vi "Dashboard Main1920x1080fixed.vi"() -> ()   [LabVIEW 2025]
uses:
  <vilib>/event_ctls.llb/eventvkey.ctl
  DashBoardGlobals.vi
  <vilib>/Rock Robotics/Network Tables/NT Read Numeric Array.vi
  <vilib>/Rock Robotics/WPI/Dashboard/WPI_DashboardLogging Global.vi
panel:
  in  "TCP":refnum<k5>
  out "Vision/Cam4Orientation":dbl caption="Cam 1 Yaw" format="%11.2f"
  out "Vision/Cam4Z":dbl caption="Cam 1 Z" format="%11.2f"
  out "Vision/Cam4Y":dbl caption="Cam 1 Y" format="%11.2f"
  out "Vision/Cam4Count":dbl caption="Cam1 Count" format="%13.0f"
  out "Vision/Cam4X":dbl caption="Cam 1 X" format="%11.2f"
  out "Vision/Cam3Orientation":dbl caption="Cam 1 Yaw" format="%11.2f"
  out "Vision/Cam3Z":dbl caption="Cam 1 Z" format="%11.2f"
  out "Vision/Cam3Y":dbl caption="Cam 1 Y" format="%11.2f"
  out "Vision/Cam3Count":dbl caption="Cam1 Count" format="%13.0f"
  out "Vision/Cam3X":dbl caption="Cam 1 X" format="%11.2f"
  out "Vision/Cam2Orientation":dbl caption="Cam 1 Yaw" format="%11.2f"
  out "Vision/Cam2Z":dbl caption="Cam 1 Z" format="%11.2f"
  out "Vision/Cam2Y":dbl caption="Cam 1 Y" format="%11.2f"
  out "Vision/Cam2Count":dbl caption="Cam1 Count" format="%13.0f"
  out "Vision/Cam2X":dbl caption="Cam 1 X" format="%11.2f"
  out "Vision/Cam1Orientation":dbl caption="Cam 1 Yaw" format="%11.2f"
  out "Vision/Cam1Z":dbl caption="Cam 1 Z" format="%11.2f"
  out "Vision/Cam1Y":dbl caption="Cam 1 Y" format="%11.2f"
  out "Vision/Cam1Count":dbl caption="Cam1 Count" format="%13.0f"
  out "Vision/Cam1X":dbl caption="Cam 1 X" format="%11.2f"
  out "NT Connection":bool
  out "Mode":T1(ring)=enum."Auto Disabled"
  out "BelowLeftCamBackground":bool
  in  "Camera Settings Right":T2={"Frame Rate"=30, "Compression"=30, "Size"=1, "DB Camera Config"=FALSE} {"Frame Rate" scale=1.0..30.0; "Compression" scale=100.0..-1.0; "Size" items=["640x480", "320x240", "160x120"]}
  in  "Camera Name Right":string(combo)="No Camera Selection"
  out "Camera Perf":string
  in  "Camera Settings":T2={"Frame Rate"=30, "Compression"=30, "Size"=1, "DB Camera Config"=FALSE} {"Frame Rate" scale=1.0..30.0; "Compression" scale=100.0..-1.0; "Size" items=["640x480", "320x240", "160x120"]}
  in  "Rec Mode":enum32{"Stop", "Record", "Playback"}(radio)
  out "Robot IP":string
  out "Image Message":string="Timeout in Camera Communications"
  in  "Dashboard Tab":T3(tab)
  out "MotorChart R":cluster{"Numeric":dbl, "Numeric":dbl}(graph)
  out "MotorChart L":cluster{"Numeric":dbl, "Numeric":dbl}(graph)
  out "MotorSliders R":cluster{"MotorSlide1":dbl, "MotorSlide2":dbl} {"MotorSlide2" scale=-1.0..1.0 scale format="%#_2e"; "MotorSlide1" scale=-1.0..1.0 scale format="%#_2e"}
  out "MotorSliders L":cluster{"MotorSlide1":dbl, "MotorSlide2":dbl} {"MotorSlide2" scale=-1.0..1.0 scale format="%#_2e"; "MotorSlide1" scale=-1.0..1.0 scale format="%#_2e"}
  out "JS1 Z":dbl(slide) scale=-1.0..1.0 scale format="%#_2e"
  out "JS1 Graph":cluster{"X":dbl, "Y":dbl}[](graph)
  out "JS1 Buttons":T4
  out "JS2 Z":dbl(slide) scale=-1.0..1.0 scale format="%#_2e"
  out "JS2 Graph":cluster{"X":dbl, "Y":dbl}[](graph)
  out "JS2 Buttons":T4
  out "Gyro":dbl(knob) scale=0.0..360.0
  out "Right Camera Perf":cluster{"Bandwidth (Mbps)":dbl, "FPS":dbl}
  out "Camera Image Right":T5(plugin-control)
  out "TurretLauncher/LauncherOn":bool caption="Launcher On"
  out "TurretLauncher/LauncherManual":bool caption="Manual"
  out "TurretLauncher/LauncherSpeed2":dbl caption="Motor 2 Speed" format="%11.0f"
  out "TurretLauncher/LauncherSpeed1":dbl caption="Motor 1 Speed" format="%11.0f"
  out "TurretLauncher/LauncherSpeedActual":dbl caption="Average Speed RPM" format="%11.0f"
  out "TurretLauncher/LauncherMotorDmd":dbl caption="Motor Dmd" format="%11.2f"
  out "TurretLauncher/LauncherTargetSpeed":dbl caption="Desired Speed RPM" format="%11.0f"
  out "TurretLauncher/SpeedOnTarget":bool caption="On Target"
  out "Teleop/GoClimb":bool caption="GO CLIMB"
  out "Teleop/FieldOriented":bool caption="Field Oriented"
  out "MatchSystem/isRed":bool caption="Is Red"
  out "MatchSystem/isBlue":bool caption="Is Blue"
  out "TurretLauncher/TurretManualMode":bool caption="Manual"
  out "TurretLauncher/TurretEncoderRotation":dbl caption="Pos Deg" format="%12.1f"
  out "TurretLauncher/OnTarget":bool caption="On Target"
  out "TurretLauncher/TurretMotorDmd":dbl caption="Motor Output" format="%11.2f"
  out "TurretLauncher/TurretDesiredAngle":dbl caption="Pos Dmd Deg" format="%12.1f"
  out "TurretLauncher/TurretclockwiseLimitSwitch":bool caption="CW Limit"
  out "TurretLauncher/TurretcounterclockwiseLimitSwitch":bool caption="CCW Limit"
  out "IntakeSystem/IntakeAngleMotorDmd":dbl caption="Pos Motor Dmd" format="%11.2f"
  out "IntakeSystem/IntakeAngleTarget":dbl caption="Position Dmd Deg" format="%12.1f"
  out "IntakeSystem/IntakeMotorRPM":dbl caption="Intake RPM" format="%12.1f"
  out "IntakeSystem/IntakeMotorOut":dbl caption="Intake Motor Dmd" format="%11.2f"
  out "IntakeSystem/EncoderRotation":dbl caption="Position Act Deg" format="%12.1f"
  out "IntakeSystem/IntakeLimitIsPressed":bool caption="LowLimitSwitch"
  out "IntakeSystem/IntakeIsExtended":bool caption="Extended"
  out "Supervisory/Mode":string caption="Mode"
  out "AutoSystem/StepTime":dbl caption="Step Time" format="%11.2f"
  out "Auto Selector":string caption="Name"
  out "AutoSystem/Step":T6(ring) caption="Cmd Name"
  out "AutoSystem/function":string caption="Function"
  out "AutoSystem/Parm2":dbl caption="Parm 2" format="%11.2f"
  out "AutoSystem/Parm1":dbl caption="Parm 1" format="%11.2f"
  out "AutoSystem/Timeout":dbl caption="Time out Sec" format="%11.2f"
  out "AutoSystem/Parm3":dbl caption="Parm 3" format="%11.2f"
  out "AutoSystem/Step":dbl caption="Cmd" format="%13.0f"
  out "TrajectorySystem/done":bool caption="Done"
  out "TrajectorySystem/ElapsedTrajTime":dbl caption="Elapsed Time" format="%12.1f"
  out "TrajectorySystem/rotErr":dbl caption="Rotational Error" format="%11.2f"
  out "TrajectorySystem/yErr":dbl caption="Y Error" format="%11.2f"
  out "TrajectorySystem/timeLengthOfTrajectory":dbl caption="Total Time" format="%12.1f"
  out "TrajectorySystem/xErr":dbl caption="X Error" format="%11.2f"
  out "TrajectorySystem/onTarget":bool caption="On Target"
  out "SwerveDrive/omegaActual":dbl caption="Vel Rot" format="%11.2f"
  out "SwerveDrive/vyActual":dbl caption="Vel Y" format="%12.1f"
  out "SwerveDrive/vyTarget":dbl caption="Vel Y Dmd" format="%12.1f"
  out "SwerveDrive/vxActual":dbl caption="Vel X" format="%12.1f"
  out "SwerveDrive/vxTarget":dbl caption="Vel X Dmd" format="%12.1f"
  out "SwerveDrive/GyroYaw":dbl caption="Gyro Yaw" format="%12.1f"
  out "SwerveDrive/GyroRoll":dbl caption="Gyro Roll" format="%12.1f"
  out "SwerveDrive/omegaTarget":dbl caption="Vel Rot Dmd" format="%11.2f"
  out "SwerveDrive/GyroPitch":dbl caption="Gyro Pitch" format="%12.1f"
  out "SwerveDrive/GyroConnected":bool caption="Gyro Connected"
  out "FeederSystem/FeederRPM":dbl caption="Speed RPM" format="%12.1f"
  out "FeederSystem/FeederOutput":dbl caption="Motor Dmd" format="%11.2f"
  out "FeederSystem/FeederState":bool caption="Feeder On"
  out "AgitatorSystem/AgitatorRPM":dbl caption="Speed  RPM" format="%12.1f"
  out "AgitatorSystem/AgitatorOutput":dbl caption="Motor Dmd" format="%11.2f"
  out "AgitatorSystem/AgitatorState":bool caption="Agitator On"
  in  "Select Auto":string(combo)="Select Autonomous ..."
  out "Odometry/Rotation_position":dbl caption="Rotation Rad" format="%11.2f"
  out "Odometry/Y_position":dbl caption="Y Pos M" format="%11.2f"
  out "Odometry/execElapsedTime":dbl caption="Elapsed Time" format="%9.3f"
  out "Odometry/X_position":dbl caption="X Pos M" format="%11.2f"
  in  "Test Slider":dbl(slide) scale=0.0..100.0 scale format="%#_3g"
  in  "On/Off":bool caption="Solenoid"
  in  "Test Name":u16(ring) items=["Select the test to run..."]
  in  "Test Tree":string(tree)
  in  "Motor":cluster{"Value":dbl, "Enable":bool} {"Value" scale=-1.0..1.0 scale format="%#_3g"}
  out "Progress":T7 {"Test Progress" scale=0.0..100.0}
  in  "Rev/Fwd":cluster{"Forward":bool, "Reverse":bool}
  in  "Test Ring":u16(ring) items=["Monochrome", "Color"]
  in  "CheckList":i32(listbox)
  out "Tree":string(tree)
  out "Camera Image":T5(plugin-control)
  out "Background":bool
  in  "Camera Name":string(combo)="No Camera Selection"
  # "VISION"
  # "Cam 1"
  # "Cam 2"
  # "Cam 3"
  # "Cam 4"
  # "Count"
  # "X"
  # "Y"
  # "Z"
  # "Yaw"
  # "HW"
  # "HW"
  # "Drive Motors"
  # "Front"
  # "Right"
  # "Left"
  # "Back"
  # "Joysticks"
  # "LAUNCHER"
  # "TELEOP"
  # "MATCH"
  # "TURRET"
  # "INTAKE"
  # "SUPERVISORY"
  # "AUTO"
  # "TRAJECTORY"
  # "DRIVE"
  # "FEEDER"
  # "AGITATOR"
  # "ODOMETRY"
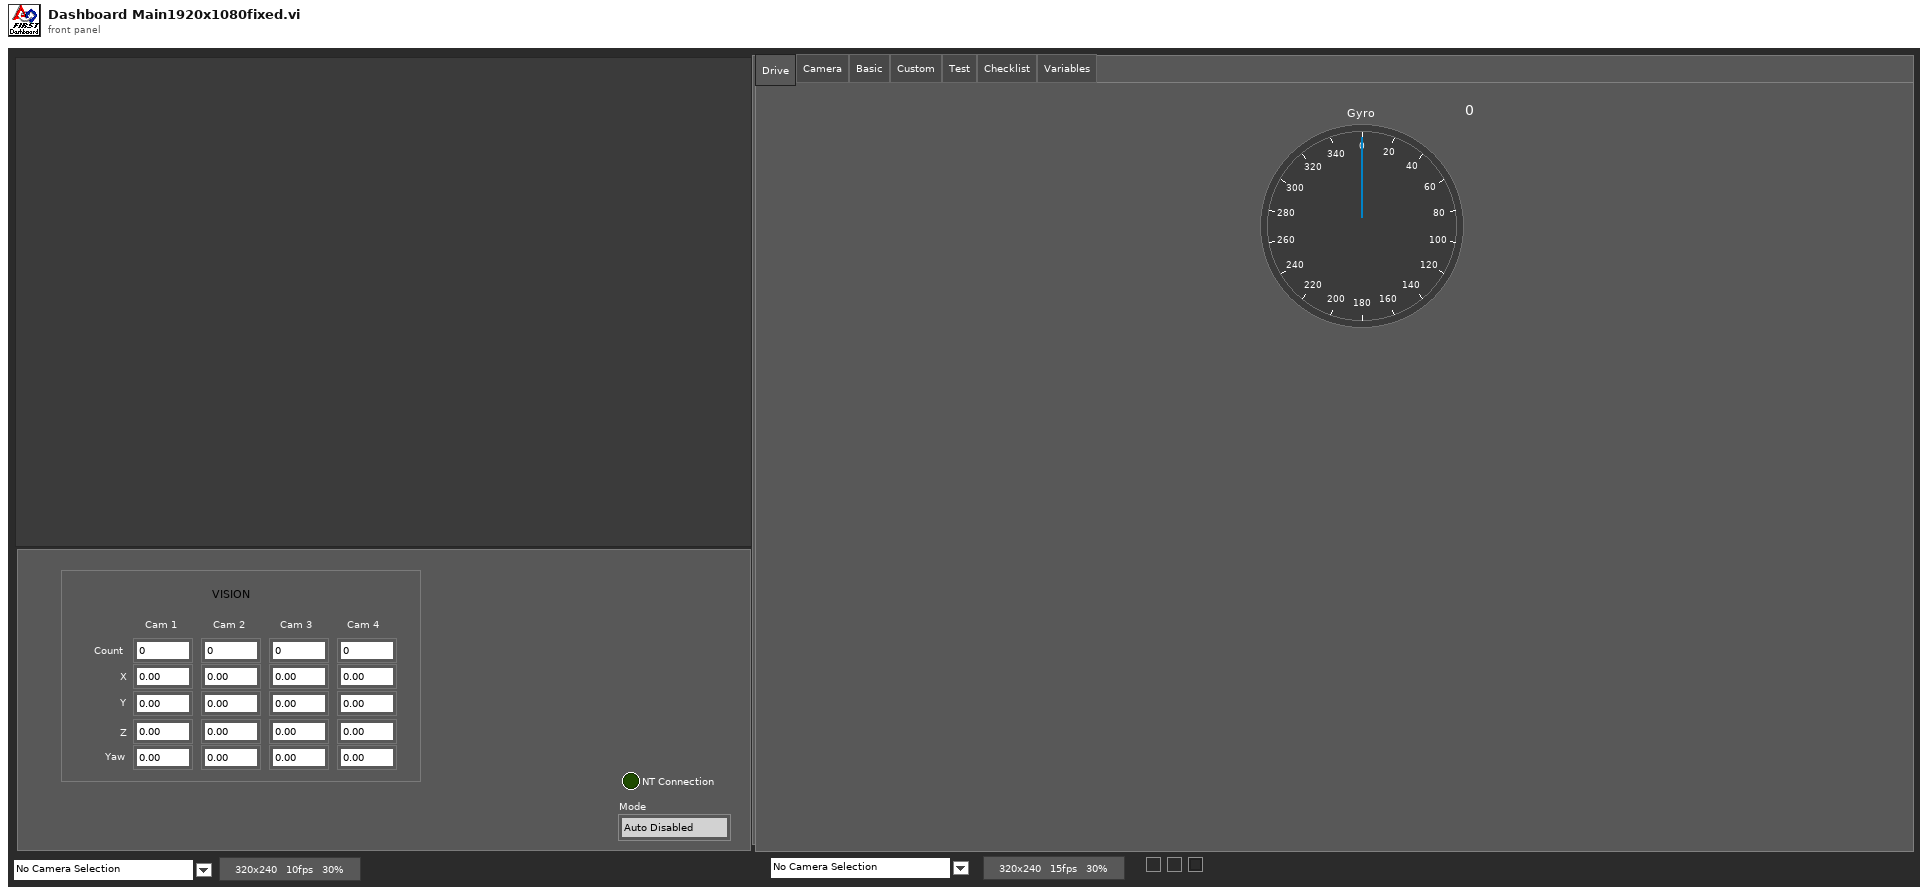
[diagram p1: front panel]
types:
  T1 = enum8{"Tele-Op Disabled", "Tele-Op Enabled", "Auto Disabled", "Auto Enabled", "Test Disabled", "Test Enabled", "Disconnected", "No Code", "E-Stop"}
  T2 = cluster{"Frame Rate":i32, "Compression":i32, "Size":u16, "DB Camera Config":bool}
  T3 = enum32{"Drive", "Camera", "Basic", "Custom", "Test", "Checklist", "Variables"}
  T4 = cluster{bool, bool, bool, bool, bool, bool, bool, bool, bool, bool, bool, bool}
  T5 = typedef "IMAQ Image.ctl" = refnum<image>
  T6 = enum16{"Drive Straight", "Drive Spin", "Follow Abs Traj", "Follow Rel Traj", "Wait", "Follow Abs Traj w/Event", "Follow Rel Traj w/Event", "Collect", "Shoot", "Balls To Alliance", "Climb", "Descend", "Unknown"}
  T7 = cluster{"Test Progress":u8, "Test Progress Text":string}
  T8 = cluster{"Save Path":path, "Interval (s)":dbl, "Keep":i32}
  T9 = enum32{"Drive", "Camera", "Basic", "Custom", "Test", "Commands", "Checklist", "Variables"}
  T10 = typedef "Image Type" = u32
  T11 = cluster{"Error Strings":string, "Disable Counts":cluster{u16, u16}, "Rail Faults":cluster{u16, u16, u16}, "Robot IP":string, "DB Mode":u8, "Event Info":cluster{"Name":string, "Type":u8, "Number":u16, "Replay":u8}}
  T12 = cluster{"Storage":cluster{"Disk Free":u64, "RAM Block":u32, "RAM free":u32}, "CPU Utilization":cluster{"CPU % ISR":sgl, "CPU % Time Crit":sgl, "CPU % Timed Str":sgl, "CPU % High":sgl, "CPU % Above":sgl, "CPU % Normal":sgl, "CPU % Low":sgl}, "CAN":cluster{"% Bus Utilization":sgl, "Bus Off Cnt":u32, "TX_FIFO Full Cnt":u32, "Receive Error Cnt":u8, "Transmit Error Cnt":u8}, "HID":cluster{"HID Outputs":u32, "Rumble Low":u16, "Rumble High":u16}[]}
  T13 = cluster{"Status bits":cluster{"Test Mode":bool, "Autonomous":bool, "Enabled":bool, "Code Start":bool, "Brownout":bool, "Reserved 2":bool, "Reserved 3":bool, "E-Stop":bool}, "Code Trace":cluster{"Disabled":bool, "TeleOp":bool, "Auto":bool, "Test":bool}, "Controller Type":enum16{"unknown", "cRIO", "roboRio"}, "Code?":enum16{"unknown", "noCode", "code"}, "Battery V":dbl}
  T14 = cluster{"Control Bits":cluster{"TestMode":bool, "Autonomous":bool, "Enabled":bool, "FMS Present":bool, bool, bool, bool, "E-Stop":bool}, "Team Station ":u8, "Countdown":sgl, "Joystick Values":cluster{"Axes":dbl[], "Buttons":bool[], "POVs":i16[]}[]}
  T15 = cluster{"Axes":dbl[], "Buttons":bool[], "POVs":i16[]}[]
  T16 = cluster{"Axes":dbl[], "Buttons":bool[], "POVs":i16[]}
  T17 = cluster{"Buttons[0]":bool, "Buttons[1]":bool, "Buttons[2]":bool, "Buttons[3]":bool, "Buttons[4]":bool, "Buttons[5]":bool, "Buttons[6]":bool, "Buttons[7]":bool, "Buttons[8]":bool, "Buttons[9]":bool, "Buttons[10]":bool, "Buttons[11]":bool}
  T18 = cluster{"Camera Image":refnum<vi>, "Dashboard Tab":refnum<vi>, "Background":refnum<vi>, "Rec Mode":refnum<vi>, "Test Slider":refnum<vi>, "On/Off ":refnum<vi>, "Test Ring":refnum<vi>, "Rev/Fwd":refnum<vi>, "Test Name":refnum<vi>, "Motor":refnum<vi>, "Progress":refnum<vi>, "CheckList":refnum<vi>, "Tree":refnum<vi>, "Test Tree":refnum<vi>, "Camera Settings":refnum<vi>, "Camera Name":refnum<vi>, "Camera Perf":refnum<vi>, "Camera Settings Right":refnum<vi>, "Camera Name Right":refnum<vi>, "Camera Image Right":refnum<vi>}
  T19 = cluster{"Global Rectangle":i32[], "Contours":cluster{"Contour Type":u32, "ROI Type":u32, "Points":i32[]}[]}
  T20 = cluster{"Camera Name":string, string, "Saved DB Images Info":cluster{"Save Path":path, "Interval (s)":dbl, "Keep":i32}}
  T21 = cluster{"Camera Name Right":string, string, "Saved DB Images Info":cluster{"Save Path":path, "Interval (s)":dbl, "Keep":i32}}
  T22 = cluster{"Operation":enum16{"Update", "Clear"}, "Color Box":u32}[]
  T23 = typedef "eventvkey.ctl" = enum16{"ASCII", "Enter", "Return", "Shift", "Ctrl", "Alt", "Cmd", "Opt", "Caps", "NumLock", "Clear", "Break", "Up", "Down", "Left", "Right", "Insert", "Delete", "Home", "End", "PageUp", "PageDown", "Escape", "Help", "Pause", "ScrollLock", "F1", "F2", "F3", "F4", "F5", "F6", "F7", "F8", "F9", "F10", "F11", "F12", "F13", "F14", "F15", "F16", "F17", "F18", "F19", "F20", "F21", "F22", "F23", "F24", "Play", "VolumeUp", "VolumeDown", "Mute", "Two Byte Char"}
  T24 = cluster{"Image Size":bool, "Image Type":bool, "Pixel Value":bool, "ROI Information":bool, "Zoom Factor":bool}
  T25 = cluster{"Operation":enum16{"Update", "Clear"}, "Color Box":u32}
  T26 = cluster{"Shift":bool, "Ctrl":bool, "Alt":bool, "Cmd":bool, "Opt":bool}
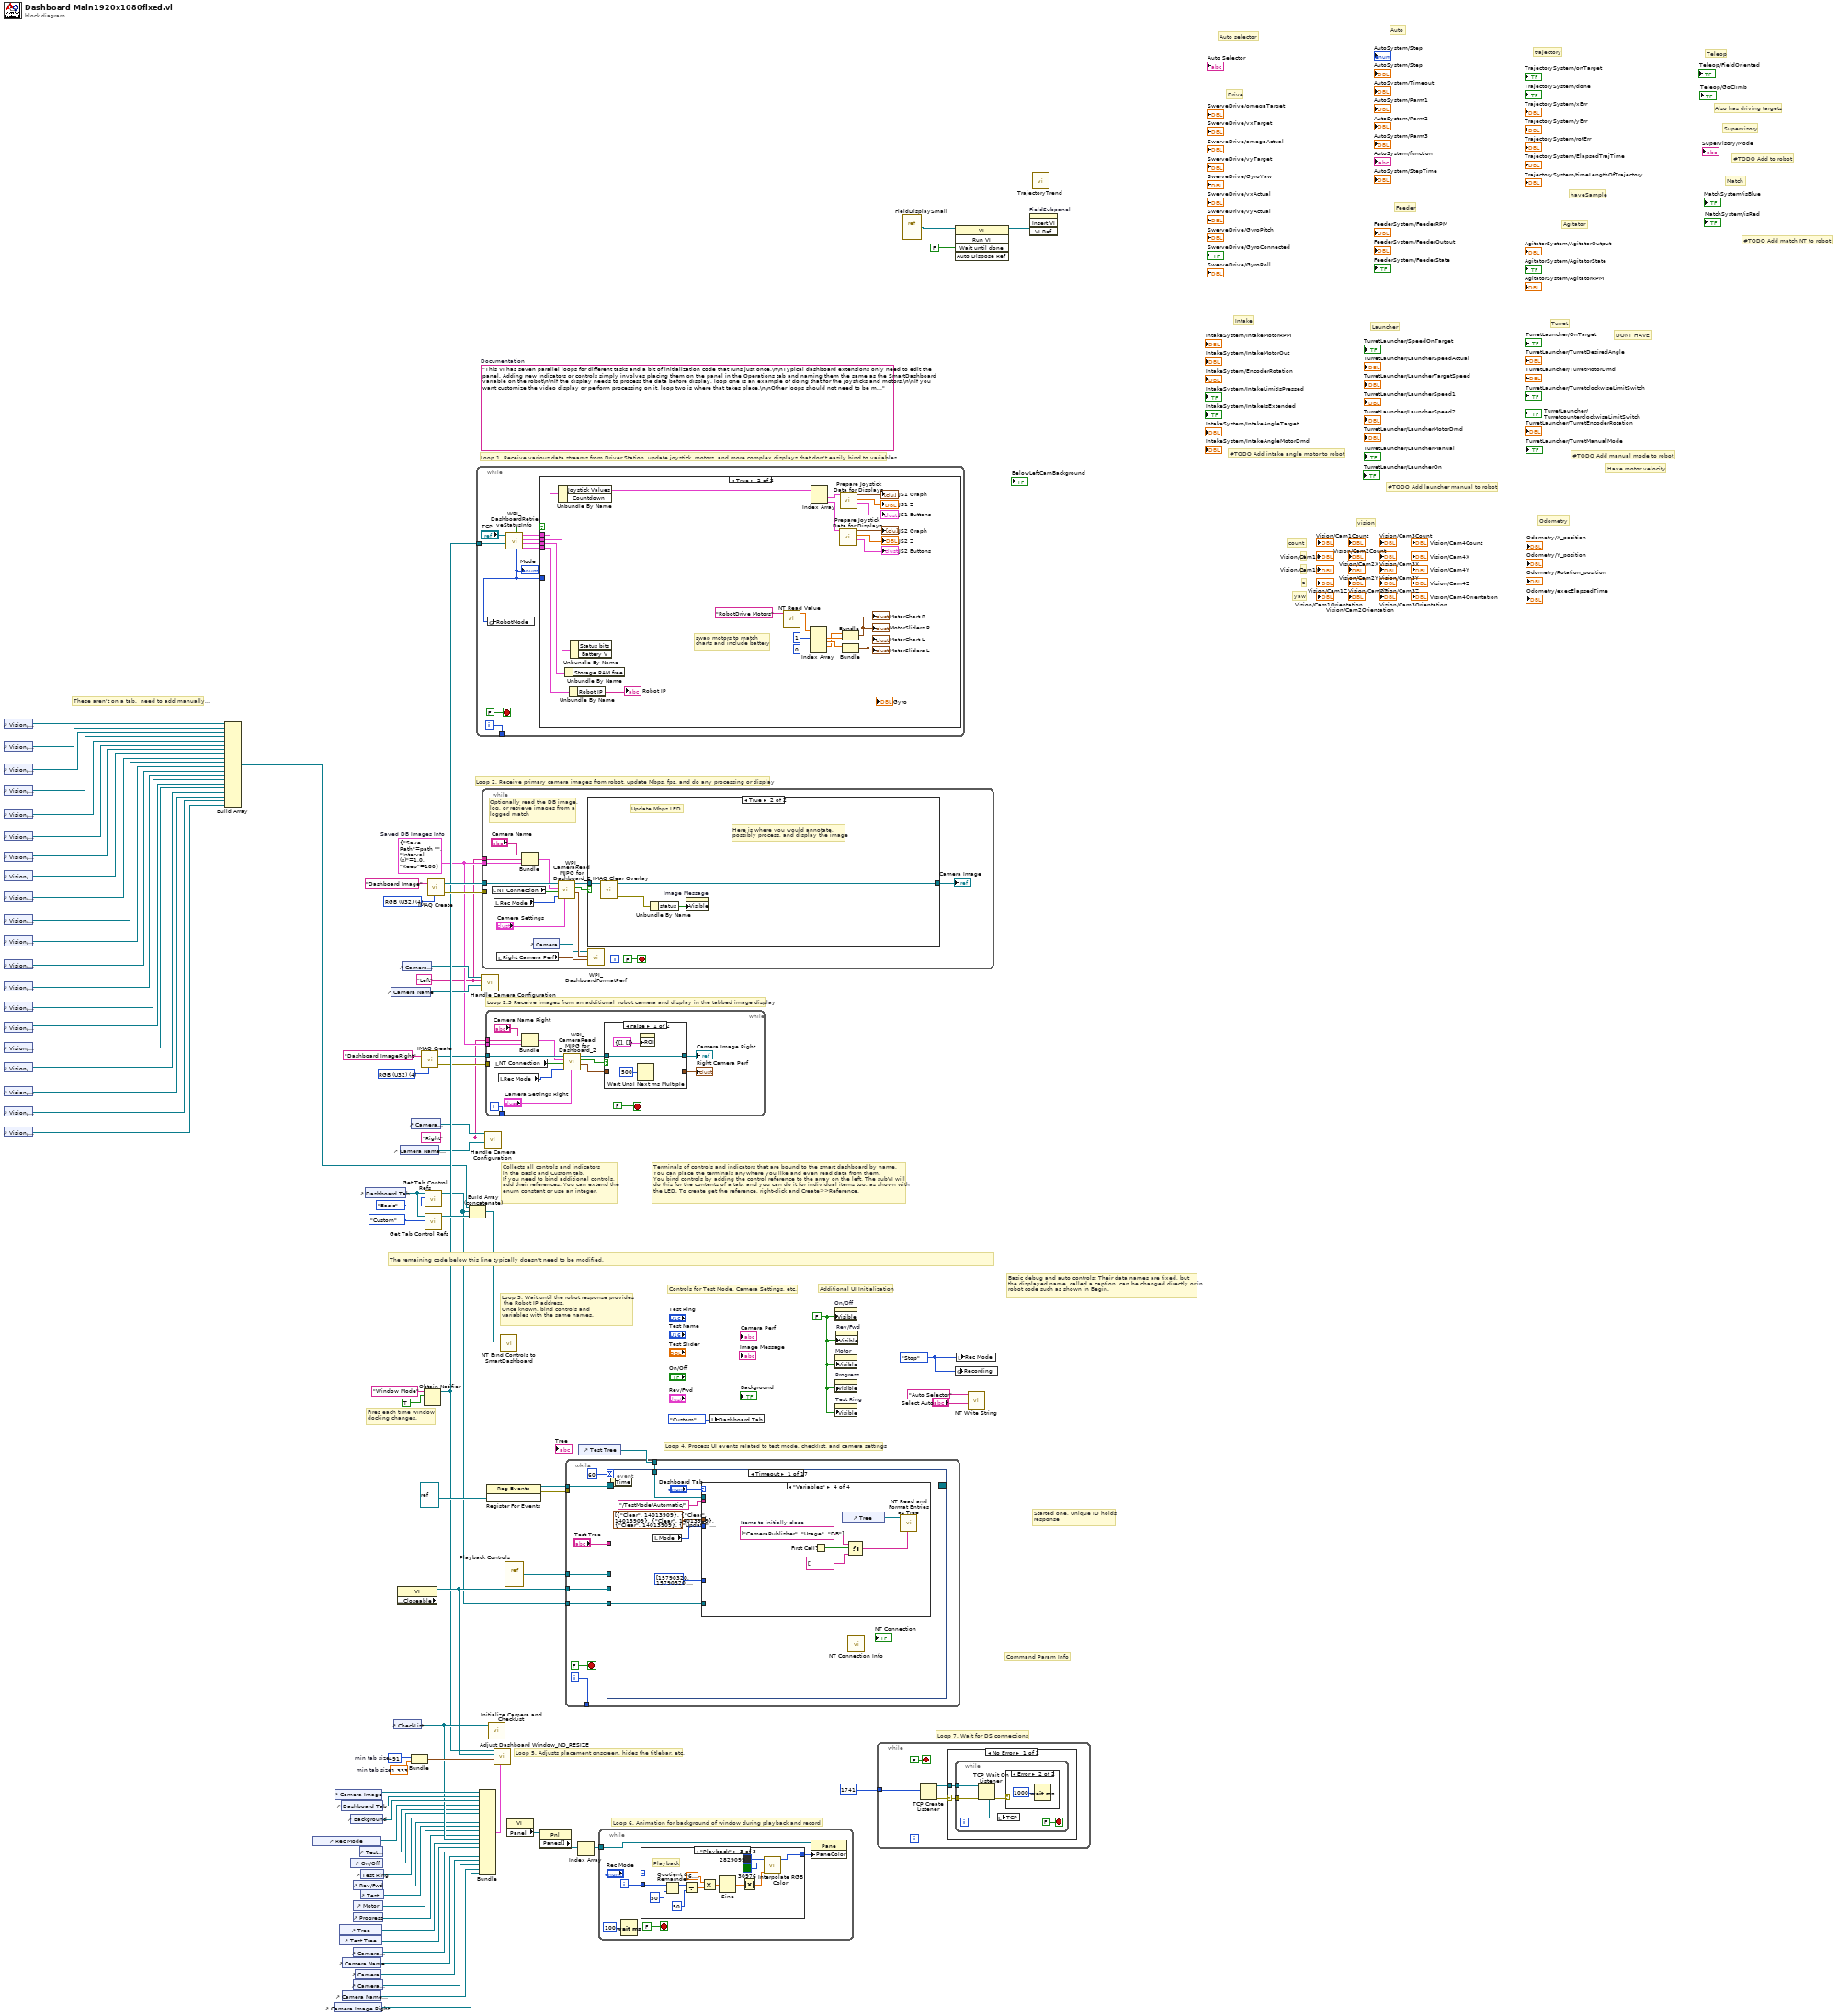
[diagram p0: block diagram]
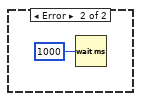
[diagram p4: hidden frame]
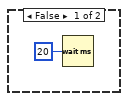
[diagram p5: hidden frame]
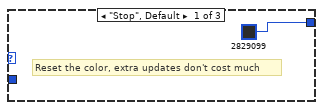
[diagram p6: hidden frame]
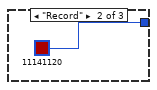
[diagram p7: hidden frame]
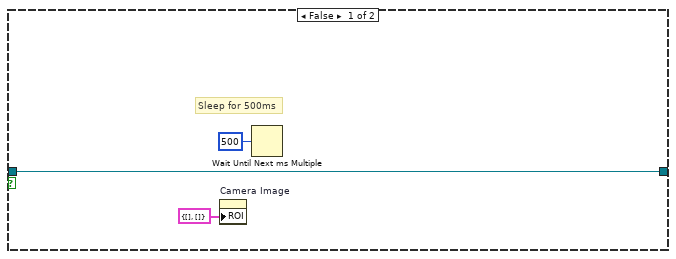
[diagram p8: hidden frame]
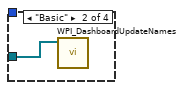
[diagram p10: hidden frame]
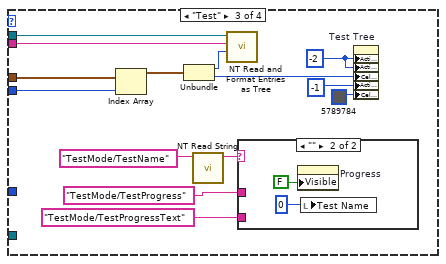
[diagram p11: hidden frame]
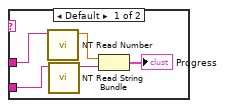
[diagram p12: hidden frame]
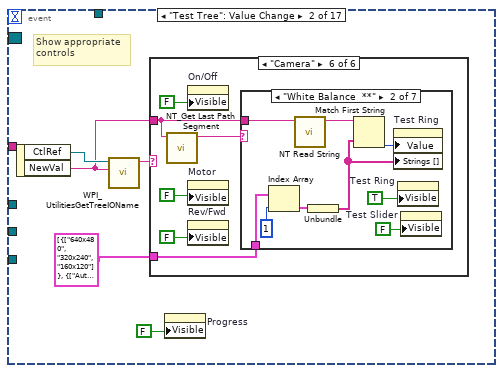
[diagram p13: hidden frame]
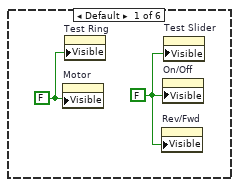
[diagram p14: hidden frame]
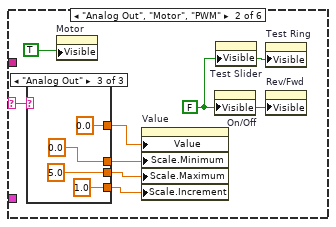
[diagram p15: hidden frame]
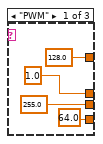
[diagram p16: hidden frame]
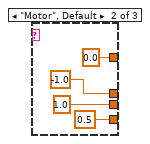
[diagram p17: hidden frame]
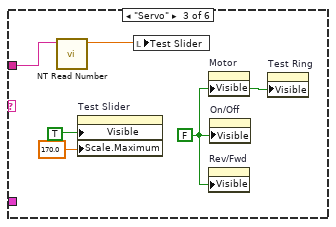
[diagram p18: hidden frame]
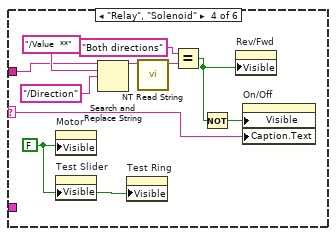
[diagram p19: hidden frame]
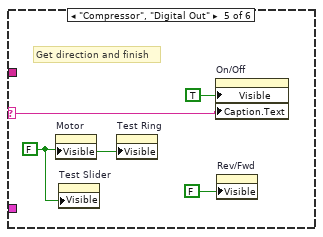
[diagram p20: hidden frame]
diagram:
  w28 = T8 {"Save Path"=path "", "Interval (s)"=1.0, "Keep"=180}  # Saved DB Images Info
  w27 = "Right"
  w26 = "Left"
  w38 = T10 4 items=["Grayscale (U8)", "Grayscale (I16)", "Grayscale (SGL)", "Complex (CSG)", "RGB (U32)", "HSL (U32)", "RGB (U64)"] ("Image Type")
  w66 = 491  # min tab size
  w65 = 1.333  # min tab size
  w73 = enum32{"Stop", "Record", "Playback"}."Stop" ("Rec Mode")
  w50 = FALSE ("Visible")
  (unwired) "This VI has seven parallel loops for different tasks and a bit of initialization code that runs just once.\n\nTypical dashboard extensions only need to edit the panel. Adding new indicators or controls simply involves placing them on the panel in the Operations tab and naming them the same as the SmartDashboard variable on the robot\n\nIf the display needs to process the data before display, loop one is an example of doing that for the joysticks and motors.\n\nIf you want customize the video display or perform processing on it, loop two is where that takes place.\n\nOther loops should not need to be modified. They are pretty standard, and document the task they perform."  # Documentation
  w87 = T10 4 items=["Grayscale (U8)", "Grayscale (I16)", "Grayscale (SGL)", "Complex (CSG)", "RGB (U32)", "HSL (U32)", "RGB (U64)"] ("Image Type")
  # "#TODO Add launcher manual to robot"
  # "#TODO Add to robot"
  # "#TODO Add match NT to robot"
  # "Match"
  # "Supervisory"
  # "#TODO Add manual mode to robot"
  # "Have motor velocity"
  # "DONT HAVE"
  # "haveSample"
  # "Also has driving targets"
  # "Teleop"
  # "Odometry"
  # "#TODO Add intake angle motor to robot"
  # "Auto selector"
  # "Drive"
  # "These aren't on a tab.  need to add manually..."
  # "Auto"
  # "trajectory"
  # "Feeder"
  # "Agitator"
  # "Intake"
  # "Turret"
  # "yaw"
  # "z"
  # "y"
  # "x"
  # "count"
  # "vision"
  # "Launcher"
  # "Loop 2.5 Receive images from an additional  robot camera and display in the tabbed image display"
  # "Command Param Info"
  # "Started one, Unique ID holds\nresponse"
  # "Loop 7. Wait for DS connections"
  # "Basic debug and auto controls: Their data names are fixed, but\nthe displayed name, called a caption, can be changed directly or in\nrobot code such as shown in Begin."
  # "Controls for Test Mode, Camera Settings, etc."
  # "Additional UI Initialization"
  # "Loop 6. Animation for background of window during playback and record"
  # "Fires each time window\ndocking changes."
  # "Collects all controls and indicators\nin the Basic and Custom tab.\nIf you need to bind additional controls,\nadd their references. You can extend the\nenum constant or use an integer."
  # "The remaining code below this line typically doesn't need to be modified."
  # "Loop 4. Process UI events related to test mode, checklist, and camera settings"
  # "Terminals of controls and indicators that are bound to the smart dashboard by name.\nYou can place the terminals anywhere you like and even read data from them.\nYou bind controls by adding the control reference to the array on the left. The subVI will\ndo this for the contents of a tab, and you can do it for individual items too, as shown with\nthe LED. To create get the reference, right-click and Create>>Reference."
  # "Loop 3. Wait until the robot response provides\n the Robot IP address.\nOnce known, bind controls and\nvariables with the same names."
  # "Loop 5. Adjusts placement onscreen, hides the titlebar, etc."
  # "Loop 1. Receive various data streams from Driver Station, update joystick, motors, and more complex displays that don't easily bind to variables."
  # "Loop 2. Receive primary camera images from robot, update Mbps, fps, and do any processing or display"
  n1 = control-ref of="Vision/Cam1Count"() -> (w21:refnum<vi>)
  n2 = control-ref of="Vision/Cam1X"() -> (w20:refnum<vi>)
  n3 = control-ref of="Vision/Cam1Y"() -> (w19:refnum<vi>)
  n4 = control-ref of="Vision/Cam1Z"() -> (w18:refnum<vi>)
  n5 = control-ref of="Vision/Cam1Orientation"() -> (w17:refnum<vi>)
  n6 = control-ref of="Vision/Cam2Count"() -> (w16:refnum<vi>)
  n7 = control-ref of="Vision/Cam2X"() -> (w15:refnum<vi>)
  n8 = control-ref of="Vision/Cam2Y"() -> (w14:refnum<vi>)
  n9 = control-ref of="Vision/Cam2Z"() -> (w13:refnum<vi>)
  n10 = control-ref of="Vision/Cam2Orientation"() -> (w12:refnum<vi>)
  n11 = control-ref of="Vision/Cam3Count"() -> (w11:refnum<vi>)
  n12 = control-ref of="Vision/Cam3X"() -> (w10:refnum<vi>)
  n13 = control-ref of="Vision/Cam3Y"() -> (w9:refnum<vi>)
  n14 = control-ref of="Vision/Cam3Z"() -> (w8:refnum<vi>)
  n15 = control-ref of="Vision/Cam3Orientation"() -> (w7:refnum<vi>)
  n16 = control-ref of="Vision/Cam4Count"() -> (w6:refnum<vi>)
  n17 = control-ref of="Vision/Cam4X"() -> (w5:refnum<vi>)
  n18 = control-ref of="Vision/Cam4Y"() -> (w4:refnum<vi>)
  n19 = control-ref of="Vision/Cam4Z"() -> (w3:refnum<vi>)
  n20 = control-ref of="Vision/Cam4Orientation"() -> (w2:refnum<vi>)
  n21 = Build Array(w21, w20, w19, w18, w17, w16, w15, w14, w13, w12, w11, w10, w9, w8, w7, w6, w5, w4, w3, w2) -> (w1:refnum<vi>[])
  n22 = control-ref of="Rec Mode"() -> (w56:refnum<vi>)
  n23 = control-ref of="Camera Image Right"() -> (w31:refnum<vi>)
  n24 = control-ref of="Camera Image"() -> (w68:refnum<vi>)
  n25 = control-ref of="Tree"() -> (w60:refnum<vi>)
  n26 = control-ref of="Test Tree"() -> (w59:refnum<vi>)
  n27 = control-ref of="Dashboard Tab"() -> (w67:refnum<vi>)
  n28 = control-ref of="Camera Name"() -> (w44:refnum<vi>)
  n29 = control-ref of="Camera Name Right"() -> (w32:refnum<vi>)
  n30 = control-ref of="Background"() -> (w63:refnum<vi>)
  n31 = control-ref of="On/Off"() -> (w54:refnum<vi>)
  n32 = control-ref of="Progress"() -> (w51:refnum<vi>)
  n33 = control-ref of="Camera Settings"() -> (w45:refnum<vi>)
  n34 = control-ref of="Camera Settings Right"() -> (w33:refnum<vi>)
  n35 = control-ref of="Rev/Fwd"() -> (w52:refnum<vi>)
  n36 = control-ref of="Motor"() -> (w57:refnum<vi>)
  n37 = control-ref of="Camera Perf"() -> (w43:refnum<vi>)
  n38 = control-ref of="Test Slider"() -> (w55:refnum<vi>)
  n39 = control-ref of="Test Ring"() -> (w53:refnum<vi>)
  n40 = control-ref of="Test Name"() -> (w58:refnum<vi>)
  n41 = control-ref of="Dashboard Tab"() -> (w71:refnum<vi>)
  n42 = control-ref of="Camera Name"() -> (w46:refnum<vi>)
  n43 = control-ref of="CheckList"() -> (w61:refnum<vi>)
  n44 = property class="VI" props=["Front Panel.Closeable"]() -> (reference out=w72:refnum<vi>)  [unwired: 2 in, 2 out]
  n45 = control-ref of="Camera Name Right"() -> (w34:refnum<vi>)
  n46 = control-ref of="Camera Settings"() -> (w47:refnum<vi>)
  n47 = control-ref of="Camera Settings Right"() -> (w35:refnum<vi>)
  n48 = Bundle("min tab size"=w66, "min tab size"=w65) -> (w64:cluster{"min tab size":i32, "min tab size":dbl})  [unwired: 1 in]
  n49 = call "IMAQ Create"("Image Name"="Dashboard ImageRight", "Image Type"=w38) -> ("New Image"=w37:T5, "error out"=w36:errorcluster)  [unwired: 2 in, 1 out]
  n50 = Obtain Notifier(name (unnamed)="Window Mode", notification data type=TRUE) -> (notifier out=w49:refnum<notifier>)  [unwired: 2 in, 2 out]
  n51 = call <vilib>:"Get Tab Control Refs.vi"("Page Index"=T9."Basic" ("Dashboard Tab"), "TabControl in"=w71) -> ("ControlsOnPage"=w42:refnum<vi>[])  [unwired: 9 in]
  n52 = call <vilib>:"Get Tab Control Refs.vi"("Page Index"=T9."Custom" ("Dashboard Tab"), "TabControl in"=w71) -> ("ControlsOnPage"=w70:refnum<vi>[])  [unwired: 9 in]
  n53 = call "IMAQ Create"("Image Name"="Dashboard Image", "Image Type"=w87) -> ("New Image"=w85:T5, "error out"=w84:errorcluster)  [unwired: 2 in, 1 out]
  n54 = Build Array (concatenate)(w1, w42, w70) -> (w69:refnum<vi>[])
  n55 = while {
    tunnel: [w96] -> _
    tunnel: w49 -> [w89]
    i -> [w96]
    stop <- FALSE stop-if-true
    n56 = call <vilib>:"WPI_DashboardRetrieveStatusInfo.vi"("Window Mode Notifier"=w89, "TCP Cnx"="TCP") -> ("Power and Errors"=w91:T11, "Robot Metrics"=w94:T12, "Status Info"=w95:T13, "Control Info"=w92:T14, "Robot Mode"=w88:T1, "Process?"=w93:bool)  [unwired: 4 in]
    "Mode" <- w88
    n57 = global write "DashBoardGlobals.vi" "RobotMode"(w88) -> ()
    n58 = case shown="True" w93 {
      tunnel: w95 -> [_ w122]
      tunnel: w94 -> [_ w121]
      tunnel: w92 -> [_ w120]
      tunnel: w91 -> [_ w119]
      tunnel: w88 -> [_ _]
      frame False {
        n59 = Wait (ms)(milliseconds to wait=u32 20) -> ()  [unwired: 1 out]
      }
      frame True {
        # "swap motors to match\ncharts and include battery"
        n60 = Unbundle By Name(w120) -> ("Joystick Values"=w110:T15)  [unwired: 1 out]
        n61 = Unbundle By Name(w121) -> ()  [unwired: 1 out]
        n62 = Unbundle By Name(w119) -> ("Robot IP"=→"Robot IP":string)
        n63 = Unbundle By Name(w122) -> ()  [unwired: 2 out]
        n64 = call-poly <vilib>:"NT Read Value.vi"("name"="RobotDrive Motors" ("Name")) -> ("value"=w100:dbl[])  [unwired: 8 in, 2 out]
        n65 = Index Array(array=w100, index #1=1, index #4=0) -> (element #1=w114:dbl, element #2=w115:dbl, element #3=w113:dbl, element #4=w118:dbl)  [unwired: 2 in]
        n66 = Index Array(array=w110) -> (element #1=w109:T16, element #2=w105:T16)  [unwired: 2 in]
        n67 = call "Prepare Joystick Data for Displays.vi"("Joystick Values"=w105) -> ("Buttons"=→"JS2 Buttons":T17, "Z Axis"=→"JS2 Z":dbl, "Cartesian Data"=→"JS2 Graph":cluster{"X axis":dbl, "X axis":dbl}[])  [unwired: 8 in]
        n68 = call "Prepare Joystick Data for Displays.vi"("Joystick Values"=w109) -> ("Buttons"=→"JS1 Buttons":T17, "Z Axis"=→"JS1 Z":dbl, "Cartesian Data"=→"JS1 Graph":cluster{"X axis":dbl, "X axis":dbl}[])  [unwired: 8 in]
        n69 = Bundle("Numeric"=w113, "Numeric"=w114) -> (→"MotorChart R" →"MotorSliders R":cluster{"Numeric":dbl, "Numeric":dbl})  [unwired: 1 in]
        n70 = Bundle("Numeric"=w115, "Numeric"=w118) -> (→"MotorChart L" →"MotorSliders L":cluster{"Numeric":dbl, "Numeric":dbl})  [unwired: 1 in]
      }
    }
  }
  n71 = Bundle("Camera Image"=w68, "Dashboard Tab"=w67, "Background"=w63, "Rec Mode"=w56, "Test Slider"=w55, "On/Off"=w54, "Test Ring"=w53, "Rev/Fwd"=w52, "Test Name"=w58, "Motor"=w57, "Progress"=w51, "CheckList"=w61, "Tree"=w60, "Test Tree"=w59, "Camera Settings"=w45, "Camera Name"=w44, "Camera Perf"=w43, "Camera Settings Right"=w33, "Camera Name Right"=w32, "Camera Image Right"=w31) -> (w62:T18)  [unwired: 1 in]
  n72 = call "Handle Camera Configuration.vi"("CameraNameRef"=w46, "Display Name"=w26, "ClusterRef"=w47) -> ()  [unwired: 9 in]
  n73 = while {
    tunnel: w85 -> [w136]
    tunnel: w84 -> [_]
    tunnel: w28 -> [w129]
    tunnel: w26 -> [w126]
    stop <- FALSE stop-if-true
    # "Optionally read the DB image,\nlog, or retrieve images from a\nlogged match"
    n74 = local read "NT Connection"() -> (w130:bool)
    n75 = local read "Rec Mode"() -> (w133:enum32{"Stop", "Record", "Playback"})
    n76 = local read "Right Camera Perf"() -> (w124:cluster{"Bandwidth (Mbps)":dbl, "FPS":dbl})
    n77 = Bundle("Camera Name"="Camera Name", w126, "Saved DB Images Info"=w129) -> (w128:T20)  [unwired: 1 in]
    n78 = control-ref of="Camera Perf"() -> (w123:refnum<vi>)
    n79 = call <vilib>:"WPI_CameraRead MJPG for Dashboard_2.vi"("Camera Settings"="Camera Settings", "Rec Mode"=w133, "NT Connection"=w130, "Capture Info"=w128, "Image in"=w136) -> ("perf info"=w125:cluster{"Bandwidth (Mbps)":dbl, "fps":dbl}, "Active"=w134:bool, "Image\\ out"=w135:T5)  [unwired: 4 in]
    n80 = case shown="True" w134 {
      tunnel: w135 -> [w139 w142]
      tunnel: [w139 w141] -> w131
      frame False {
        # "Sleep for 500ms"
        n81 = property on="Camera Image" class="ImageControl"("ROI"=T19 {"Global Rectangle"=[], "Contours"=[]}) -> ()  [unwired: 2 in, 2 out]
        n82 = Wait Until Next ms Multiple(millisecond multiple=u32 500) -> ()  [unwired: 1 out]
      }
      frame True {
        # "Here is where you would annotate,\npossibly process, and display the image"
        # "Update Mbps LED"
        n83 = call "IMAQ Clear Overlay"("Image"=w142) -> ("error out"=w143:errorcluster, "Image Out"=w141:T5)  [unwired: 2 in, 7 out]
        n84 = Unbundle By Name(w143) -> ("status"=w144:bool)
        n85 = property on="Image Message" class="Str"("Visible"=w144) -> ()  [unwired: 2 in, 2 out]
      }
    }
    "Camera Image" <- w131
    n86 = call <vilib>:"WPI_DashboardFormatPerf.vi"("Right Camera Perf"=w124, "Performance"=w125, "String in"=w123) -> ()  [unwired: 9 in]
  }
  n87 = call "Handle Camera Configuration.vi"("CameraNameRef"=w34, "Display Name"=w27, "ClusterRef"=w35) -> ()  [unwired: 9 in]
  n88 = while {
    tunnel: w37 -> [w159]
    tunnel: w36 -> [_]
    tunnel: [w154] -> _
    tunnel: w28 -> [w150]
    tunnel: w27 -> [w147]
    i -> [w154]
    stop <- FALSE stop-if-true
    n89 = local read "NT Connection"() -> (w151:bool)
    n90 = local read "Rec Mode"() -> (w158:enum32{"Stop", "Record", "Playback"})
    n91 = Bundle("Camera Name Right"="Camera Name Right", w147, "Saved DB Images Info"=w150) -> (w149:T21)  [unwired: 1 in]
    n92 = call <vilib>:"WPI_CameraRead MJPG for Dashboard_2.vi"("Camera Settings"="Camera Settings Right", "Rec Mode"=w158, "NT Connection"=w151, "Capture Info"=w149, "Image in"=w159) -> ("perf info"=w145:cluster{"Bandwidth (Mbps)":dbl, "fps":dbl}, "Active"=w153:bool, "Image\\ out"=w156:T5)  [unwired: 4 in]
    n93 = case shown="False" w153 {
      tunnel: w156 -> [w161 w164]
      tunnel: [w161 w164] -> w152
      tunnel: [_ w163] -> w146
      tunnel: w145 -> [_ w163]
      frame False {
        n94 = Wait Until Next ms Multiple(millisecond multiple=u32 500) -> ()  [unwired: 1 out]
        n95 = property on="Camera Image Right" class="ImageControl"("ROI"=T19 {"Global Rectangle"=[], "Contours"=[]}) -> ()  [unwired: 2 in, 2 out]
      }
      frame True {
      }
    }
    "Camera Image Right" <- w152
    "Right Camera Perf" <- w146
  }
  n96 = register-events(refnum<vi> refnum) -> (reference out=w76:refnum<event-registration>, error out=w75:errorcluster)  [unwired: 2 in]
  n97 = call "Initialize Camera and CheckList.vi"("ListBox in"=w61) -> ()  [unwired: 11 in]
  n98 = call "Adjust Dashboard Window_NO_RESIZE.vi"("Sizing Refnums"=w62, "Size Constraints"=w64, "VI"=w72, "WIn Mode"=w49) -> ()  [unwired: 8 in]
  n99 = call <vilib>:"NT Bind Controls to SmartDashboard.vi"("Bound Control Refs"=w69) -> ()  [unwired: 11 in]
  n100 = vi-ref "Playback Controls.vi"() -> (w77:refnum<vi>)
  n101 = property class="VI"() -> ("Panel"=w79:refnum<vi>)  [unwired: 2 in, 2 out]
  n102 = property class="Pnl"(reference=w79) -> ("Panes[]"=w80:refnum<vi>[])  [unwired: 1 in, 2 out]
  n103 = Index Array(array=w80) -> (element=w78:refnum<vi>)  [unwired: 1 in]
  n104 = control-ref of="Test Tree"() -> (w81:refnum<vi>)
  n105 = while {
    tunnel: [w170] -> _
    tunnel: w81 -> [w169]
    tunnel: w77 -> [w168]
    tunnel: w76 -> [w167]
    tunnel: w75 -> [_]
    tunnel: w72 -> [w166]
    tunnel: w42 -> [w165]
    i -> [w170]
    stop <- FALSE stop-if-true
    n106 = event shown="[0] Timeout" {
      selector: w167 -> [_ _ _ _ _ _ _ _ _ _ _ _ _ _ _ _ _]
      dyn-events: [_ _ _ _ _ _ _ _ _ _ _ _ _ w375 _ _ _] -> _
      timeout: u32 60 ("milliseconds to wait") -> [_ _ _ _ _ _ _ _ _ _ _ _ _ _ _ _ _]
      tunnel: w169 -> [w181 _ _ _ _ _ _ _ _ _ _ _ _ _ _ _ _]
      tunnel: "Test Tree" -> [_ _ _ _ _ _ _ _ w348 w355 w356 w359 w366 _ _ _ _]
      tunnel: w168 -> [_ _ _ _ _ _ _ _ _ _ _ _ _ w377 _ w392 _]
      tunnel: w166 -> [_ _ _ _ _ _ _ _ _ _ _ _ _ w373 _ _ _]
      tunnel: w165 -> [w176 _ _ _ _ _ _ _ _ _ _ _ _ _ _ _ _]
      event Timeout {
        n107 = event-data() -> ()  [unwired: 1 in, 1 out]
        n108 = local read "Mode"() -> (w179:T1)
        n109 = case shown="\"Variables\"" "Dashboard Tab" {
          tunnel: w181 -> [_ _ w196 _]
          tunnel: "/TestMode/Automatic/" ("Name Pattern") -> [_ _ w195 _]
          tunnel: T22 [{"Operation"=enum."Clear", "Color Box"=14013909}, {"Operation"=enum."Clear", "Color Box"=14013909}, {"Operation"=enum."Clear", "Color Box"=14013909}, {"Operation"=enum."Clear", "Color Box"=14013909}, {"Operation"=enum."Update", "Color Box"=14013909}, {"Operation"=enum."Update", "Color Box"=16777215}, {"Operation"=enum."Clear", "Color Box"=14013909}, {"Operation"=enum."Clear", "Color Box"=14013909}, {"Operation"=enum."Clear", "Color Box"=14013909}] -> [_ _ w188 _]
          tunnel: w179 -> [_ _ w187 _]
          tunnel: u32[] [15790320, 15790320, 15790320, 15790320, 16777215, 16777215, 15790320, 15790320, 15790320] -> [_ _ _ _]
          tunnel: w176 -> [_ w182 _ _]
          frame "Custom", Default {
          }
          frame "Basic" {
            n110 = call <vilib>:"WPI_DashboardUpdateNames.vi"("Controls on Tab"=w182) -> ()  [unwired: 11 in]
          }
          frame "Test" {
            w194 = -2 ("Active Item:Row Number")
            n111 = Index Array(array=w188, index=w187) -> (element=w189:T25)
            n112 = Unbundle(w189) -> ("Operation"=w190:enum16{"Update", "Clear"}, "Color Box"=w191:u32)
            n113 = call <vilib>:"NT Read String.vi"("name"="TestMode/TestName" ("Name")) -> ("value"=w185:string)  [unwired: 8 in, 2 out]
            n114 = call <vilib>:"NT Read and Format Entries as Tree.vi"("Operation"=w190, "Name Pattern"=w195, "Tree Refnum"=w196) -> ()  [unwired: 7 in, 2 out]
            n115 = case shown="\"\"" w185 {
              tunnel: "TestMode/TestProgress" ("Name") -> [w198 _]
              tunnel: "TestMode/TestProgressText" ("Name") -> [w197 _]
              frame Default {
                n116 = call <vilib>:"NT Read Number.vi"("name"=w198) -> ("value"=w199:dbl)  [unwired: 8 in, 2 out]
                n117 = call <vilib>:"NT Read String.vi"("name"=w197) -> ("value"=w200:string)  [unwired: 8 in, 2 out]
                n118 = Bundle("value"=w199, "value"=w200) -> (→"Progress":cluster{"value":dbl, "value":string})  [unwired: 1 in]
              }
              frame "" {
                n119 = property on="Progress" class="Clust (strict)"("Visible"=FALSE) -> ()  [unwired: 2 in, 2 out]
                n120 = local write "Test Name"(u16 0) -> ()
              }
            }
            n121 = property on="Test Tree" class="Tree (strict)"("Active Item Row Number"=w194, "ActiveColNum"=w194, "CellBG"=w191, "Active Item Row Number"=-1 ("Active Item:Row Number"), "CellBG"=u32 5789784 ("Color Box")) -> ()  [unwired: 2 in, 2 out]
          }
          frame "Variables" {
            w206 = string[] ["CameraPublisher", "Usage", "DB"]  # Items to initially close
            n122 = First Call?() -> (First Call?: T/F=w207:bool)
            n123 = control-ref of="Tree"() -> (w208:refnum<vi>)
            n124 = Select(t=w206, s=w207, f=string[] []) -> (s? t:f=w204:string[])
            n125 = call <vilib>:"NT Read and Format Entries as Tree.vi"("Tags to  Close"=w204, "Tree Refnum"=w208) -> ()  [unwired: 8 in, 2 out]
          }
        }
        n126 = call <vilib>:"NT Connection Info.vi"() -> ("Connected"=→"NT Connection":bool)  [unwired: 11 in]
      }
      event "Test Tree": Value Change {
        # "Show appropriate\ncontrols"
        n127 = event-data() -> ("CtlRef"=w212:refnum<vi>, "NewVal"=w210:string)  [unwired: 1 in]
        n128 = call <vilib>:"WPI_UtilitiesGetTreeIOName.vi"("NewVal"=w210, "TreeControl in"=w212) -> ("I/O Name"=w213:string)  [unwired: 9 in]
        n129 = case shown="\"Camera\"" w213 {
          selector: w213 -> [_ w220 _ w242 w251 _]
          tunnel: w210 -> [_ _ w239 w241 _ w258]
          tunnel: cluster{string[]}[] [{["640x480", "320x240", "160x120"]}, {["Auto", "Fixed indoor", "Fixed outdoor 1", "Fixed outdoor 2", "Fixed fluorescent 1", "Fixed fluorescent 2", "Hold current"]}, {["Auto", "Flicker-free 50 Hz", "Flicker-free 60 Hz", "Hold current"]}, {["None", "Prioritize frame rate", "Prioritize image quality"]}, {["Monochrome", "Color"]}] -> [_ _ _ _ _ w257]
          frame Default {
            w215 = FALSE ("Visible")
            w214 = FALSE ("Visible")
            n130 = property on="Motor" class="Clust (strict)"("Visible"=w214) -> ()  [unwired: 2 in, 2 out]
            n131 = property on="Test Ring" class="Ring (strict)"("Visible"=w214) -> ()  [unwired: 2 in, 2 out]
            n132 = property on="Rev/Fwd" class="Clust (strict)"("Visible"=w215) -> ()  [unwired: 2 in, 2 out]
            n133 = property on="On/Off" class="Bool (strict)"("Visible"=w215) -> ()  [unwired: 2 in, 2 out]
            n134 = property on="Test Slider" class="Slide (strict)"("Visible"=w215) -> ()  [unwired: 2 in, 2 out]
          }
          frame "Analog Out", "Motor", "PWM" {
            w221 = FALSE ("Visible")
            n135 = case shown="\"Analog Out\"" w220 {
              tunnel: [1.0 ("Value") -1.0 ("Value") 0.0 ("Value")] -> w219
              tunnel: [255.0 ("Value") 1.0 ("Value") 5.0 ("Value")] -> w218
              tunnel: [128.0 ("Value") 0.0 ("Value") 0.0 ("Value")] -> w217
              tunnel: [64.0 ("Value") 0.5 ("Value") 1.0 ("Value")] -> w216
              frame "PWM" {
              }
              frame "Motor", Default {
              }
              frame "Analog Out" {
              }
            }
            n136 = property on="Motor" class="Clust (strict)"("Visible"=TRUE) -> ()  [unwired: 2 in, 2 out]
            n137 = property on="Value" class="Slide (strict)"("Value"=w217, "Scale.Minimum"=w219, "Scale.Maximum"=w218, "Scale.Increment"=w216) -> ()  [unwired: 2 in, 2 out]
            n138 = property on="On/Off" class="Bool (strict)"("Visible"=w221) -> ()  [unwired: 2 in, 2 out]
            n139 = property on="Test Slider" class="Slide (strict)"("Visible"=w221) -> ()  [unwired: 2 in, 2 out]
            n140 = property on="Test Ring" class="Ring (strict)"("Visible"=w221) -> ()  [unwired: 2 in, 2 out]
            n141 = property on="Rev/Fwd" class="Clust (strict)"("Visible"=w221) -> ()  [unwired: 2 in, 2 out]
          }
          frame "Servo" {
            w237 = FALSE ("Visible")
            n142 = call <vilib>:"NT Read Number.vi"("name"=w239) -> ("value"=w238:dbl)  [unwired: 8 in, 2 out]
            n143 = property on="Test Slider" class="Slide (strict)"("Visible"=TRUE, "Scale.Maximum"=170.0 ("Scale.Range:Maximum")) -> ()  [unwired: 2 in, 2 out]
            n144 = local write "Test Slider"(w238) -> ()
            n145 = property on="Motor" class="Clust (strict)"("Visible"=w237) -> ()  [unwired: 2 in, 2 out]
            n146 = property on="Rev/Fwd" class="Clust (strict)"("Visible"=w237) -> ()  [unwired: 2 in, 2 out]
            n147 = property on="On/Off" class="Bool (strict)"("Visible"=w237) -> ()  [unwired: 2 in, 2 out]
            n148 = property on="Test Ring" class="Ring (strict)"("Visible"=w237) -> ()  [unwired: 2 in, 2 out]
          }
          frame "Relay", "Solenoid" {
            w240 = FALSE ("Visible")
            n149 = property on="Motor" class="Clust (strict)"("Visible"=w240) -> ()  [unwired: 2 in, 2 out]
            n150 = property on="Test Slider" class="Slide (strict)"("Visible"=w240) -> ()  [unwired: 2 in, 2 out]
            n151 = Search and Replace String(input string=w241, search string="/Value  **", replace string="/Direction") -> (result string=w247:string)  [unwired: 5 in, 3 out]
            n152 = property on="Test Ring" class="Ring (strict)"("Visible"=w240) -> ()  [unwired: 2 in, 2 out]
            n153 = call <vilib>:"NT Read String.vi"("name"=w247) -> ("value"=w245:string)  [unwired: 8 in, 2 out]
            n154 = Equal?(x="Both directions", y=w245) -> (x = y?=w243:bool)
            n155 = Not(x=w243) -> (.not. x?=w244:bool)
            n156 = property on="Rev/Fwd" class="Clust (strict)"("Visible"=w243) -> ()  [unwired: 2 in, 2 out]
            n157 = property on="On/Off" class="Bool (strict)"("Visible"=w244, "Caption.Text"=w242) -> ()  [unwired: 2 in, 2 out]
          }
          frame "Compressor", "Digital Out" {
            w250 = FALSE ("Visible")
            # "Get direction and finish"
            n158 = property on="Motor" class="Clust (strict)"("Visible"=w250) -> ()  [unwired: 2 in, 2 out]
            n159 = property on="Test Slider" class="Slide (strict)"("Visible"=w250) -> ()  [unwired: 2 in, 2 out]
            n160 = property on="Test Ring" class="Ring (strict)"("Visible"=w250) -> ()  [unwired: 2 in, 2 out]
            n161 = property on="On/Off" class="Bool (strict)"("Visible"=TRUE, "Caption.Text"=w251) -> ()  [unwired: 2 in, 2 out]
            n162 = property on="Rev/Fwd" class="Clust (strict)"("Visible"=FALSE) -> ()  [unwired: 2 in, 2 out]
          }
          frame "Camera" {
            n163 = call <vilib>:"NT_Get Last Path Segment.vi"("String in"=w258) -> ("String out"=w259:string)  [unwired: 10 in]
            n164 = property on="On/Off" class="Bool (strict)"("Visible"=FALSE) -> ()  [unwired: 2 in, 2 out]
            n165 = property on="Motor" class="Clust (strict)"("Visible"=FALSE) -> ()  [unwired: 2 in, 2 out]
            n166 = property on="Rev/Fwd" class="Clust (strict)"("Visible"=FALSE) -> ()  [unwired: 2 in, 2 out]
            n167 = case shown="\"White Balance  **\"" w259 {
              tunnel: w258 -> [w265 w274 w283 w292 w301 _ w307]
              tunnel: w257 -> [w263 w271 w280 w289 w298 _ _]
              frame "Size  **" {
                n168 = Index Array(array=w263) -> (element=w262:cluster{string[]})  [unwired: 1 in]
                n169 = call <vilib>:"NT Read String.vi"("name"=w265) -> ("value"=w264:string)  [unwired: 8 in, 2 out]
                n170 = Unbundle(w262) -> (w260:string[])
                n171 = Match First String(2:w260, 3:w264) -> (0:w261:i32)  [unwired: 1 out]
                n172 = property on="Test Ring" class="Ring (strict)"("Value"=w261, "Strings []"=w260) -> ()  [unwired: 2 in, 2 out]
                n173 = property on="Test Ring" class="Ring (strict)"("Visible"=TRUE) -> ()  [unwired: 2 in, 2 out]
                n174 = property on="Test Slider" class="Slide (strict)"("Visible"=FALSE) -> ()  [unwired: 2 in, 2 out]
              }
              frame "White Balance  **" {
                n175 = Index Array(array=w271, index=1) -> (element=w272:cluster{string[]})
                n176 = call <vilib>:"NT Read String.vi"("name"=w274) -> ("value"=w273:string)  [unwired: 8 in, 2 out]
                n177 = Unbundle(w272) -> (w269:string[])
                n178 = Match First String(2:w269, 3:w273) -> (0:w268:i32)  [unwired: 1 out]
                n179 = property on="Test Ring" class="Ring (strict)"("Value"=w268, "Strings []"=w269) -> ()  [unwired: 2 in, 2 out]
                n180 = property on="Test Ring" class="Ring (strict)"("Visible"=TRUE) -> ()  [unwired: 2 in, 2 out]
                n181 = property on="Test Slider" class="Slide (strict)"("Visible"=FALSE) -> ()  [unwired: 2 in, 2 out]
              }
              frame "Exposure  **" {
                n182 = Index Array(array=w280, index=2) -> (element=w281:cluster{string[]})
                n183 = call <vilib>:"NT Read String.vi"("name"=w283) -> ("value"=w282:string)  [unwired: 8 in, 2 out]
                n184 = Unbundle(w281) -> (w277:string[])
                n185 = Match First String(2:w277, 3:w282) -> (0:w278:i32)  [unwired: 1 out]
                n186 = property on="Test Ring" class="Ring (strict)"("Value"=w278, "Strings []"=w277) -> ()  [unwired: 2 in, 2 out]
                n187 = property on="Test Ring" class="Ring (strict)"("Visible"=TRUE) -> ()  [unwired: 2 in, 2 out]
                n188 = property on="Test Slider" class="Slide (strict)"("Visible"=FALSE) -> ()  [unwired: 2 in, 2 out]
              }
              frame "Exposure Priority  **" {
                n189 = Index Array(array=w289, index=3) -> (element=w290:cluster{string[]})
                n190 = call <vilib>:"NT Read String.vi"("name"=w292) -> ("value"=w291:string)  [unwired: 8 in, 2 out]
                n191 = Unbundle(w290) -> (w286:string[])
                n192 = Match First String(2:w286, 3:w291) -> (0:w287:i32)  [unwired: 1 out]
                n193 = property on="Test Ring" class="Ring (strict)"("Value"=w287, "Strings []"=w286) -> ()  [unwired: 2 in, 2 out]
                n194 = property on="Test Ring" class="Ring (strict)"("Visible"=TRUE) -> ()  [unwired: 2 in, 2 out]
                n195 = property on="Test Slider" class="Slide (strict)"("Visible"=FALSE) -> ()  [unwired: 2 in, 2 out]
              }
              frame "Color Enable  **" {
                n196 = Index Array(array=w298, index=4) -> (element=w299:cluster{string[]})
                n197 = call <vilib>:"NT Read String.vi"("name"=w301) -> ("value"=w300:string)  [unwired: 8 in, 2 out]
                n198 = Unbundle(w299) -> (w295:string[])
                n199 = Match First String(2:w295, 3:w300) -> (0:w296:i32)  [unwired: 1 out]
                n200 = property on="Test Ring" class="Ring (strict)"("Value"=w296, "Strings []"=w295) -> ()  [unwired: 2 in, 2 out]
                n201 = property on="Test Ring" class="Ring (strict)"("Visible"=TRUE) -> ()  [unwired: 2 in, 2 out]
                n202 = property on="Test Slider" class="Slide (strict)"("Visible"=FALSE) -> ()  [unwired: 2 in, 2 out]
              }
              frame Default {
                n203 = property on="Test Ring" class="Ring (strict)"("Visible"=FALSE) -> ()  [unwired: 2 in, 2 out]
                n204 = property on="Test Slider" class="Slide (strict)"("Visible"=FALSE) -> ()  [unwired: 2 in, 2 out]
              }
              frame "Brightness  **", "Color Level  **", "Compression  **", "FPS  **", "Sharpness  **" {
                n205 = call <vilib>:"NT Read Number.vi"("name"=w307) -> ("value"=w306:dbl)  [unwired: 8 in, 2 out]
                n206 = local write "Test Slider"(w306) -> ()
                n207 = property on="Test Ring" class="Ring (strict)"("Visible"=FALSE) -> ()  [unwired: 2 in, 2 out]
                n208 = property on="Test Slider" class="Slide (strict)"("Visible"=TRUE, "Scale.Maximum"=100.0 ("Scale.Range:Maximum")) -> ()  [unwired: 2 in, 2 out]
              }
            }
          }
        }
        n209 = property on="Progress" class="Clust (strict)"("Visible"=FALSE) -> ()  [unwired: 2 in, 2 out]
      }
      event "Test Name": Mouse Enter {
        # "Populate the ring with the list of tests"
        n210 = event-data() -> ()  [unwired: 1 in, 1 out]
        n211 = call <vilib>:"NT Read String Array.vi"("name"="TestMode/TestList" ("Name")) -> ("value"=w314:string[])  [unwired: 8 in, 2 out]
        n212 = Build Array (concatenate)("Select the test to run...", w314) -> (w313:string[])
        n213 = property on="Test Name" class="Ring (strict)"("Strings []"=w313) -> ()  [unwired: 2 in, 2 out]
      }
      event "Test Name": Value Change {
        w315 = FALSE ("Visible")
        # "Tell the robot the test name to run"
        n214 = event-data() -> ("NewVal"=w319:u16)  [unwired: 1 in]
        n215 = property on="Test Name" class="Ring (strict)"() -> ("Strings []"=w320:string[])  [unwired: 2 in, 2 out]
        n216 = local write "Progress"(T7 {"Test Progress"=0, "Test Progress Text"=""} ("Progress")) -> ()
        n217 = Index Array(array=w320, index=w319) -> (element=w318:string)
        n218 = call <vilib>:"NT Write String.vi"("value"=w318, "name"="TestMode/TestName" ("Name")) -> ()  [unwired: 9 in, 1 out]
        n219 = property on="Progress" class="Clust (strict)"("Visible"=TRUE) -> ()  [unwired: 2 in, 2 out]
        n220 = property on="Motor" class="Clust (strict)"("Visible"=w315) -> ()  [unwired: 2 in, 2 out]
        n221 = property on="Test Slider" class="Slide (strict)"("Visible"=w315) -> ()  [unwired: 2 in, 2 out]
        n222 = property on="On/Off" class="Bool (strict)"("Visible"=w315) -> ()  [unwired: 2 in, 2 out]
        n223 = property on="Rev/Fwd" class="Clust (strict)"("Visible"=w315) -> ()  [unwired: 2 in, 2 out]
        n224 = property on="Test Ring" class="Ring (strict)"("Visible"=w315) -> ()  [unwired: 2 in, 2 out]
      }
      event "Select Auto": Mouse Enter {
        # "Populate the combo box with the list of autonomous options"
        n225 = event-data() -> ()  [unwired: 1 in, 1 out]
        n226 = call <vilib>:"NT Read String Array.vi"("name"="Auto List" ("Name")) -> ("value"=w322:string[])  [unwired: 8 in, 2 out]
        n227 = property on="Select Auto" class="CmbBox"("Strings[]"=w322) -> ()  [unwired: 2 in, 2 out]
      }
      event "Select Auto": Value Change {
        # "User modified the Auto Selection. Write to NT variable so robot knows."
        n228 = event-data() -> ("NewVal"=w324:string)  [unwired: 1 in]
        n229 = call <vilib>:"NT Write String.vi"("value"=w324, "name"="Auto Selector" ("Name")) -> ()  [unwired: 9 in, 1 out]
      }
      event "CheckList": Double Click {
        # "Shift clears all"
        # "Update symbols on the listbox"
        n230 = event-data() -> ("PlatMods.Shift"=w326:bool, "Row"=w328:i32)  [unwired: 1 in]
        n231 = case shown="True" w326 {
          tunnel: w328 -> [w332 _]
          tunnel: 1 -> [w331 _]
          frame False {
            n232 = property on="CheckList" class="LstBox (strict)"() -> ("Item Symbols"=w330:i32[])  [unwired: 2 in, 2 out]
            n233 = Replace Array Subset(array=w330, new element=w331, index=w332) -> (w329:i32[])
            n234 = property on="CheckList" class="LstBox (strict)"("Item Symbols"=w329) -> ()  [unwired: 2 in, 2 out]
          }
          frame True {
            w333 = 0 ("Top Row")
            n235 = property on="CheckList" class="LstBox (strict)"() -> ("Number of Rows"=w335:u32)  [unwired: 2 in, 2 out]
            n236 = Initialize Array(0, w335) -> (w334:i32[])
            n237 = property on="CheckList" class="LstBox (strict)"("Top Row"=w333, "Value"=w333, "Item Symbols"=w334) -> ()  [unwired: 2 in, 2 out]
          }
        }
      }
      event "CheckList": Key Down {
        # "Update symbols on the listbox\nLeft and right keys check and uncheck"
        n238 = event-data() -> ("VKey"=w338:T23)  [unwired: 1 in]
        n239 = case shown="\"Left\", \"Right\"" w338 {
          selector: w338 -> [w343 _]
          tunnel: eventvkey."Left" ("VKey") -> [w341 _]
          frame "Left", "Right" {
            n240 = Equal?(x=w341, y=w343) -> (x = y?=w342:bool)
            n241 = Select(t=0, s=w342, f=1) -> (s? t:f=w344:i32)
            n242 = property on="CheckList" class="LstBox (strict)"() -> ("Item Symbols"=w347:i32[])  [unwired: 2 in, 2 out]
            n243 = Replace Array Subset(array=w347, new element=w344, index="CheckList") -> (w346:i32[])
            n244 = property on="CheckList" class="LstBox (strict)"("Item Symbols"=w346) -> ()  [unwired: 2 in, 2 out]
          }
          frame Default {
          }
        }
      }
      event "Motor.Enable": Value Change {
        # "When the test mode otor enable helper is set, update that\ntree row item's value"
        n245 = event-data() -> ("NewVal"=w352:bool)  [unwired: 1 in]
        n246 = Unbundle("Motor") -> ("Value"=w351:dbl)  [unwired: 1 out]
        n247 = Select(t=w351, s=w352, f=0.0) -> (s? t:f=w349:dbl)
        n248 = call <vilib>:"NT Write Number.vi"("value"=w349, "name"=w348) -> ()  [unwired: 9 in, 1 out]
      }
      event "Test Slider": Value Change {
        # "When the test mode slider helper is set, update that\ntree row item's value"
        n249 = event-data() -> ("NewVal"=w354:dbl)  [unwired: 1 in]
        n250 = call <vilib>:"NT Write Number.vi"("value"=w354, "name"=w355) -> ()  [unwired: 9 in, 1 out]
      }
      event "On/Off": Value Change {
        # "When the test mode on/off helper value is set, update that\ntree row item's value"
        n251 = event-data() -> ("NewVal"=w358:bool)  [unwired: 1 in]
        n252 = Boolean To (0,1)(Boolean=w358) -> (0, 1=w357:i16)
        n253 = call <vilib>:"NT Write Number.vi"("value"=w357, "name"=w356) -> ()  [unwired: 9 in, 1 out]
      }
      event "Rev/Fwd": Value Change {
        # "When the test mode helper value for relays is set, update that\ntree row item's value"
        n254 = event-data() -> ("NewVal.Forward"=w365:bool, "NewVal.Reverse"=w364:bool)  [unwired: 1 in]
        n255 = Boolean To (0,1)(Boolean=w365) -> (0, 1=w361:i16)
        n256 = Boolean To (0,1)(Boolean=w364) -> (0, 1=w363:i16)
        n257 = Negate(x=w363) -> (-x=w362:i16)
        n258 = Add(x=w361, y=w362) -> (x+y=w360:i16)
        n259 = call <vilib>:"NT Write Number.vi"("value"=w360, "name"=w359) -> ()  [unwired: 9 in, 1 out]
      }
      event "Test Ring": Value Change {
        # "When a test mode helper value is selected from the ring,\nset the tree item's variable to the string value"
        n260 = event-data() -> ("NewVal"=w368:u16)  [unwired: 1 in]
        n261 = property on="Test Ring" class="Ring (strict)"() -> ("Strings []"=w369:string[])  [unwired: 2 in, 2 out]
        n262 = Index Array(array=w369, index=w368) -> (element=w367:string)
        n263 = call <vilib>:"NT Write String.vi"("value"=w367, "name"=w366) -> ()  [unwired: 9 in, 1 out]
      }
      event "Rec Mode": Value Change {
        # "Update globals for recording mode and path to read log from.\nClear when logging and let NetworkTables set path for vision to\nuse."
        n264 = event-data() -> ("NewVal"=w378:enum32{"Stop", "Record", "Playback"})  [unwired: 1 in]
        n265 = global write "WPI_DashboardLogging Global.vi" "Logging Filename"(path "") -> ()
        n266 = global write "WPI_DashboardLogging Global.vi" "Recording"(w378) -> ()
        n267 = case shown="\"Playback\"" w378 {
          tunnel: w377 -> [_ w380 w388]
          tunnel: [_ _ w387] -> w375
          tunnel: [_ _ w386] -> _
          tunnel: w373 -> [_ _ w384]
          tunnel: cluster{i32, i32} {-250, 170} -> [_ _ w383]
          tunnel: [_ _ T24 {"Image Size"=TRUE, "Image Type"=TRUE, "Pixel Value"=TRUE, "ROI Information"=TRUE, "Zoom Factor"=FALSE} ("Image Information Shown:All Elements")] -> w370
          tunnel: [_ _ TRUE ("Zoom Factor")] -> w371
          frame Default {
          }
          frame "Stop", "Record" {
            # "Place Window too"
            n268 = invoke class="VI" method="FP.Close"(reference=w380) -> (reference out=w379:refnum<vi>)  [unwired: 2 in, 2 out]
            n269 = invoke class="VI" method="Abort VI"(reference=w379) -> ()  [unwired: 2 in, 3 out]
          }
          frame "Playback" {
            n270 = call "Open Playback Panel.vi"("Offset"=w383, "DB VI Ref"=w384, "Playback in"=w388) -> ("Playback out"=w385:refnum<vi>)  [unwired: 8 in]
            n271 = register-events(w385) -> (reference out=w387:refnum<event-registration>, error out=w386:errorcluster)  [unwired: 2 in]
          }
        }
        n272 = property on="Camera Image Right" class="ImageControl"("Image Information Shown"=w370, "Image Information Visible"=w371) -> ()  [unwired: 2 in, 2 out]
        n273 = property on="Camera Image" class="ImageControl"("Image Information Shown"=w370, "Image Information Visible"=w371) -> ()  [unwired: 2 in, 2 out]
        n274 = call <vilib>:"WPI_DashboardNT Log FieldName Cache.vi"("Operation"=enum16{"Lookup/Add", "Index", "Clear"}."Clear") -> ()  [unwired: 8 in, 3 out]
      }
      event Panel Close {
        w389 = enum32{"Stop", "Record", "Playback"}."Stop" ("Rec Mode")
        # "Playback window has been closed, abort"
        n275 = event-data() -> ()  [unwired: 1 in, 4 out]
        n276 = local write "Rec Mode"(w389) -> ()
        n277 = global write "WPI_DashboardLogging Global.vi" "Recording"(w389) -> ()
      }
      event Panel Close {
        # "Abort playback window and ourself"
        n278 = event-data() -> ()  [unwired: 1 in, 4 out]
        n279 = invoke class="VI" method="FP.Close"(reference=w392) -> (reference out=w391:refnum<vi>)  [unwired: 2 in, 2 out]
        n280 = invoke class="VI" method="Abort VI"(reference=w391) -> (error out=w390:errorcluster)  [unwired: 2 in, 2 out]
        n281 = invoke class="VI" method="Abort VI"(error in=w390) -> ()  [unwired: 2 in, 3 out]
      }
      event "Tree": Double Click {
        n282 = event-data() -> ("PlatMods"=w398:T26, "Tag"=w395:string)  [unwired: 1 in]
        n283 = Unbundle(w398) -> ("Shift"=w397:bool)  [unwired: 4 out]
        n284 = String Subset(string=w395, length (rest)=1 ("length (rest)")) -> (substring=w394:string)  [unwired: 1 in]
        n285 = Not(x=w397) -> (.not. x?=w396:bool)
        n286 = case shown="\"/\"" w394 {
          tunnel: w395 -> [_ w400]
          tunnel: w396 -> [_ w399]
          frame Default {
          }
          frame "/" {
            n287 = call <vilib>:"NT Update Persistence.vi"("Persistence"=w399, "Name"=w400) -> ()  [unwired: 9 in, 1 out]
          }
        }
      }
    }
  }
  n288 = while {
    tunnel: w78 -> [w402]
    i -> [w405]
    stop <- FALSE stop-if-true
    n289 = Wait (ms)(milliseconds to wait=u32 100) -> ()  [unwired: 1 out]
    n290 = case shown="\"Playback\"" "Rec Mode" {
      tunnel: w405 -> [_ _ w420]
      tunnel: [u32 2829099 ("Base Color") u32 11141120 ("Target Color") w409] -> w401
      frame "Stop", Default {
        # "Reset the color, extra updates don't cost much"
      }
      frame "Record" {
      }
      frame "Playback" {
        # "Playback"
        n291 = Quotient & Remainder(x=w420, y=u32 50 ("milliseconds to wait")) -> (x-y*floor(x/y)=w416:u32)  [unwired: 1 out]
        n292 = Divide(x=w416, y=u32 50 ("milliseconds to wait")) -> (x/y=w413:dbl)
        n293 = Multiply(x=6.283185307179586, y=w413) -> (x*y=w418:dbl)
        n294 = Sine(x=w418) -> (sin(x)=w417:dbl)
        n295 = Absolute Value(x=w417) -> (abs(x)=w410:dbl)
        n296 = call "Interpolate RGB Color.vi"("Proportion"=w410, "Target Color"=u32 30976, "Base Color"=u32 2829099) -> ("Result Color"=w409:u32)  [unwired: 8 in]
      }
    }
    n297 = property class="Pane"(reference=w402, "PaneColor"=w401) -> ()  [unwired: 1 in, 2 out]
  }
  n298 = local write "Dashboard Tab"(T3."Custom" ("Dashboard Tab")) -> ()
  n299 = property on="On/Off" class="Bool (strict)"("Visible"=w50) -> ()  [unwired: 2 in, 2 out]
  n300 = property on="Motor" class="Clust (strict)"("Visible"=w50) -> ()  [unwired: 2 in, 2 out]
  n301 = property on="Progress" class="Clust (strict)"("Visible"=w50) -> ()  [unwired: 2 in, 2 out]
  n302 = property on="Test Ring" class="Ring (strict)"("Visible"=w50) -> ()  [unwired: 2 in, 2 out]
  n303 = property on="Rev/Fwd" class="Clust (strict)"("Visible"=w50) -> ()  [unwired: 2 in, 2 out]
  n304 = while {
    tunnel: u16 1741 ("timeout ms (25000)") -> [w422]
    stop <- FALSE stop-if-true
    n305 = TCP Create Listener(10:w422) -> (0:w421:errorcluster, 3:w423:refnum<k5>)  [unwired: 4 in, 1 out]
    n306 = case shown="No Error" w421 {
      selector: w421 -> [w425 _]
      tunnel: w423 -> [w426 _]
      frame No Error {
        n307 = while {
          tunnel: w426 -> [w429]
          tunnel: w425 -> [w428]
          stop <- FALSE stop-if-true
          n308 = TCP Wait On Listener(8:w428, 11:w429) -> (0:w430:errorcluster, 4:w431:refnum<k5>)  [unwired: 2 in, 3 out]
          n309 = local write "TCP"(w431) -> ()
          n310 = case shown="Error" w430 {
            frame No Error {
            }
            frame Error {
              n311 = Wait (ms)(milliseconds to wait=u32 1000) -> ()  [unwired: 1 out]
            }
          }
        }
      }
      frame Error {
        n312 = Wait (ms)(milliseconds to wait=u32 1000) -> ()  [unwired: 1 out]
      }
    }
  }
  n313 = vi-ref "FieldDisplaySmall.vi"() -> (w25:refnum<vi>)
  n314 = invoke class="VI" method="Run VI"(reference=w25, "Wait until done"=FALSE ("Wait Until Done")) -> (reference out=w23:refnum<vi>)  [unwired: 3 in, 4 out]
  n315 = global write "WPI_DashboardLogging Global.vi" "Recording"(w73) -> ()
  n316 = local write "Rec Mode"(w73) -> ()
  n317 = call <vilib>:"NT Write String.vi"("value"="Select Auto", "name"="Auto Selector" ("Name")) -> ()  [unwired: 9 in, 1 out]
  n318 = invoke on="FieldSubpanel" class="SubPnl" method="Insert VI"("VI Ref"=w23) -> ()  [unwired: 3 in, 4 out]
  n319 = call "TrajectoryTrend.vi"() -> ()  [unwired: 12 in]
